vi "Omit RTEXE Results.vi"(8 "error in (no error)":errorcluster, 9 "Message Data":variant, 10 "Message":string) -> (0 "error out":errorcluster)   [LabVIEW 2024, in "User Interface.lvlib"]
uses:
  User Interface.lvlib
  Support/General Type Defs/Global Data.vi
  Support/General Type Defs/General Type Definitions.lvlib
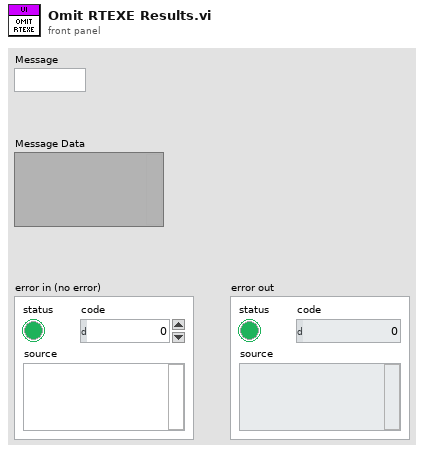
[diagram p1: front panel]
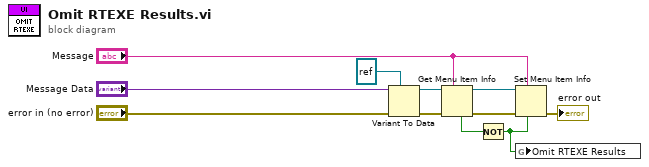
[diagram p0: block diagram]
diagram:
  n1 = Variant To Data(error in="error in (no error)", type=refnum<k9> refnum ("MenuRef"), Variant="Message Data") -> (data=w2:refnum<k9>, error out=w4:errorcluster)
  n2 = Get Menu Item Info(7:"Message", 8:w4, 11:w2) -> (0:w6:errorcluster, 3:w5:refnum<k9>, 4:w7:bool)  [unwired: 4 out]
  n3 = Not(x=w7) -> (.not. x?=w8:bool)
  n4 = Set Menu Item Info(6:w8, 7:"Message", 8:w6, 11:w5) -> (0:→"error out":errorcluster)  [unwired: 3 in, 1 out]
  n5 = global write "Global Data.vi" "Omit RTEXE Results"(w8) -> ()
